vi "RAM Diagnostics.vi"() -> (0 "error out":errorcluster, 3 "Result":bool)   [LabVIEW 2025]
doc: "Performs diagnostics on the Random Access Memory (RAM) installed on the motherboard."
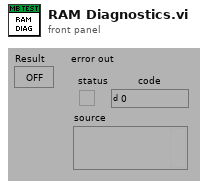
[diagram p1: front panel]
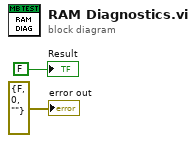
[diagram p0: block diagram]
diagram:
  "error out" <- errorcluster {"status"=FALSE, "code"=0, "source"=""} ("error out")
  "Result" <- FALSE ("PASS/FAIL Flag")
